vi "hComRegStop2013.vi"(4 "error in":errorcluster, 7 "FPGA VI Reference In":refnum<k20>) -> (0 "error out":errorcluster, 2 "Timed Out":bool, 3 "FPGA VI Reference Out":refnum<k20>)   [LabVIEW 2014]
doc: "Schreibt in das Komunikationsregister um kontinuierlichen Lesemodus zu starten."
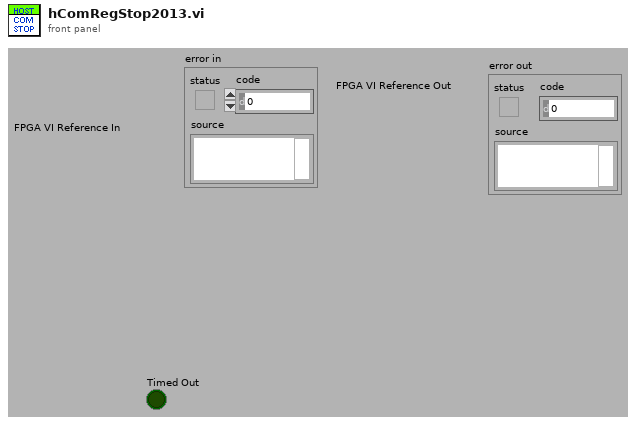
[diagram p1: front panel]
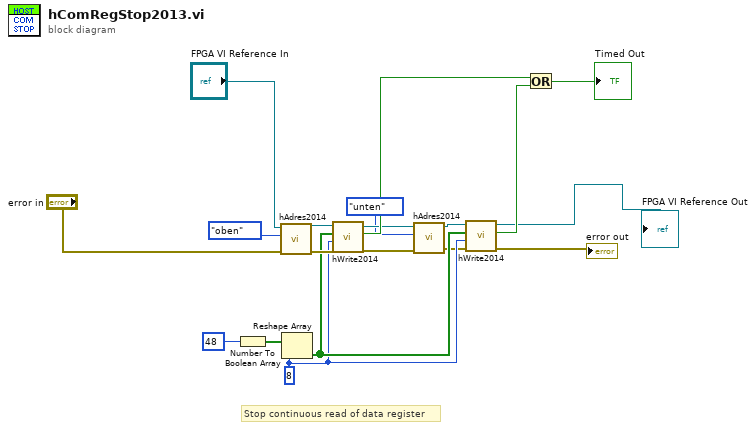
[diagram p0: block diagram]
diagram:
  w6 = u8 8
  # "Stop continuous read of data register"
  n1 = Number To Boolean Array(number=u8 48 ("t")) -> (Boolean array=w17:bool[])
  n2 = call "hAdres2014.vi"("error in"="error in", "AdressMode"=enum16{"select", "oben", "unten", "keinen"}."oben", "FPGA VI Reference In"="FPGA VI Reference In") -> ("error out"=w13:errorcluster, "FPGA VI Reference Out"=w16:refnum<k20>)  [unwired: 3 in]
  n3 = Reshape Array(w17, w6) -> (w7:bool[])
  n4 = call "hWrite2014.vi"("error in"=w13, "nbit"=w6, "Data"=w7, "FPGA VI Reference In"=w16) -> ("error out"=w9:errorcluster, "Timed Out"=w12:bool, "FPGA VI Reference Out"=w10:refnum<k20>)  [unwired: 1 in]
  n5 = call "hAdres2014.vi"("error in"=w9, "AdressMode"=enum16{"select", "oben", "unten", "keinen"}."unten", "FPGA VI Reference In"=w10) -> ("error out"=w5:errorcluster, "FPGA VI Reference Out"=w11:refnum<k20>)  [unwired: 3 in]
  n6 = call "hWrite2014.vi"("error in"=w5, "nbit"=w6, "Data"=w7, "FPGA VI Reference In"=w11) -> ("error out"=→"error out":errorcluster, "Timed Out"=w4:bool, "FPGA VI Reference Out"=→"FPGA VI Reference Out":refnum<k20>)  [unwired: 1 in]
  n7 = Or(x=w12, y=w4) -> (x .or. y?=→"Timed Out":bool)
